vi "Cannon Sensors Update.vi"(1 "Cannon Information":T1) -> (0 "Cannon Information out":T1)   [LabVIEW 2012]
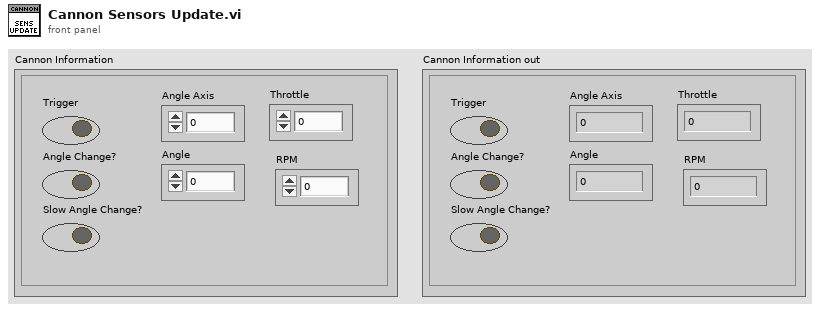
[diagram p1: front panel]
types:
  T1 = cluster{"RPM":dbl, "Trigger":bool, "Angle Axis":dbl, "Angle":dbl, "Throttle":dbl, "Slow Angle Change?":bool, "Angle Change?":bool}
  T2 = typedef "WPI_AnalogChannelDevRef.ctl" = cluster{"DevStatus":errorcluster, "Analog Module":T3, "Analog Channel":T4}
  T3 = typedef "FPGA_TypedefAnalogModule.ctl" = enum16{"Analog Module 1", "Analog Module 2"}
  T4 = typedef "FPGA_AIChannel.ctl" = enum8{"AI 1", "AI 2", "AI 3", "AI 4", "AI 5", "AI 6", "AI 7", "AI 8", "Invalid"}
  T5 = typedef "WPI_CounterDevRef.ctl" = cluster{"DevStatus":errorcluster, "CntIndex":T6}
  T6 = typedef "FPGA_CounterCtrSystemIndex.ctl" = enum8{"Ctr 0", "Ctr 1", "Ctr 2", "Ctr 3", "Ctr 4", "Ctr 5", "Ctr 6", "Ctr 7", "Invalid"}
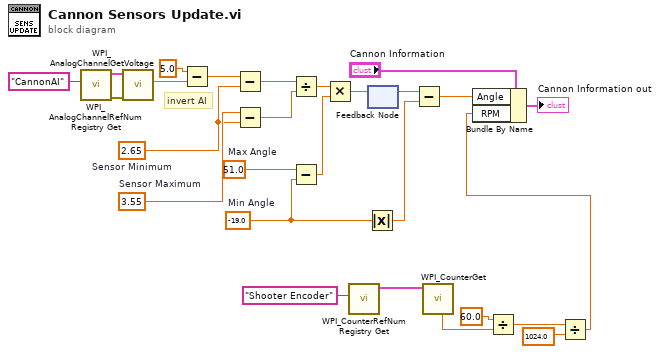
[diagram p0: block diagram]
diagram:
  w19 = 2.65  # Sensor Minimum
  w20 = 3.55  # Sensor Maximum
  w12 = 51.0  # Max Angle
  w11 = -19.0  # Min Angle
  # "invert AI"
  n1 = call <vilib>:"WPI_AnalogChannelRefNum Registry Get.vi"("refnum name"="CannonAI") -> ("error out"=w25:errorcluster, "AIDeviceRef"=w26:T2)  [unwired: 9 in]
  n2 = call <vilib>:"WPI_AnalogChannelGetVoltage.vi"("error in (no error)"=w25, "AIDeviceRef"=w26) -> ("Voltage"=w15:dbl)  [unwired: 7 in, 2 out]
  n3 = Subtract(x=5.0, y=w15) -> (x-y=w14:dbl)
  n4 = Subtract(x=w14, y=w19) -> (x-y=w17:dbl)
  n5 = Subtract(x=w20, y=w19) -> (x-y=w18:dbl)
  n6 = Divide(x=w17, y=w18) -> (x/y=w23:dbl)
  n7 = Subtract(x=w12, y=w11) -> (x-y=w24:dbl)
  n8 = Multiply(x=w23, y=w24) -> (x*y=w22:dbl)
  n9 = call <vilib>:"WPI_CounterRefNum Registry Get.vi"("refnum name"="Shooter Encoder") -> ("CounterDevRef"=w2:T5)  [unwired: 9 in, 1 out]
  n10 = Absolute Value(x=w11) -> (abs(x)=w13:dbl)
  n11 = feedback #1() -> (w21:dbl)  [unwired: 1 in]
  n12 = feedback-in #1(w22) -> ()
  n13 = Subtract(x=w21, y=w13) -> (x-y=w10:dbl)
  n14 = call <vilib>:"WPI_CounterGet.vi"("CounterDevRef in"=w2) -> ("Period (sec)"=w3:dbl)  [unwired: 5 in, 5 out]
  n15 = Divide(x=60.0, y=w3) -> (x/y=w4:dbl)
  n16 = Divide(x=w4, y=1024.0) -> (x/y=w1:dbl)
  n17 = Bundle By Name(cluster="Cannon Information", "Angle"=w10, "RPM"=w1) -> (→"Cannon Information out":T1)
